vi "Qn15_X.vi"(11 "String":string) -> (3 "Qn":dbl[](array[numeric]))   [LabVIEW 2015]
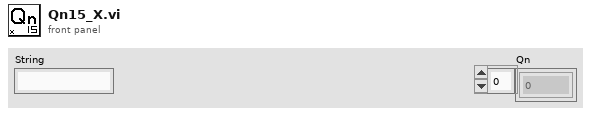
[diagram p1: front panel]
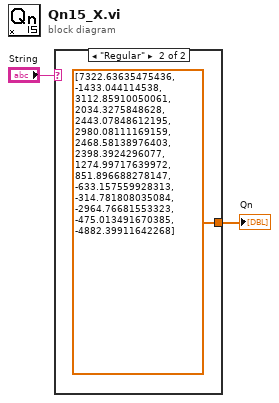
[diagram p0: block diagram]
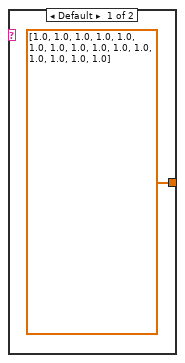
[diagram p2: hidden frame]
diagram:
  n1 = case shown="\"Regular\"" "String" {
    tunnel: [dbl[] [1.0, 1.0, 1.0, 1.0, 1.0, 1.0, 1.0, 1.0, 1.0, 1.0, 1.0, 1.0, 1.0, 1.0, 1.0] ("Qn") dbl[] [7322.63635475436, -1433.044114538, 3112.85910050061, 2034.3275848628, 2443.07848612195, 2980.08111169159, 2468.58138976403, 2398.3924296077, 1274.99717639972, 851.896688278147, -633.157559928313, -314.781808035084, -2964.76681553323, -475.013491670385, -4882.39911642268] ("Qn")] -> w2
    frame Default {
    }
    frame "Regular" {
    }
  }
  "Qn" <- w2
